vi "Action Update Ramp Rate-test-Caraya.vi"(8 "error in (no error)":errorcluster) -> (0 "error out":errorcluster)   [LabVIEW 2018]
doc: "The harness VI is executed for every test case. InstaCoverage passes the test case ID before the execution of the test case in the <b>test case ID</b> input and reads the <b>result</b> output after the execution. If the result is TRUE and no error happens during the execution, then the test case is evaluated as PASSED. If the result is false and no error happens during the execution, then the test case is evaluated as FAILED. Otherwise the test case is evaluated as ERROR.\n\nThe result of the test suite will be PASSED (FAILED) if all (at least one) test cases are PASSED (FAILED). If at least one test case in the test suite has the ERROR result, then the test suite will have ERROR result.\n\n<b>Note: </b>Don't change the connector pane of this VI.\n\nSee the Help Document for more information. (<b>Help</b> > <b>IncQuery Labs</b> > <b>InstaCoverage</b> > <b>InstaCoverage Help...</b>)"
uses:
  <vilib>/addons/_JKI Toolkits/Caraya/classes/Assert/Assert True.vi
  Libraries/Thermal Chamber Controller_DQMH/Thermal Chamber Controller_DQMH.lvlib
  <vilib>/addons/_JKI Toolkits/Caraya/classes/Test/Test.lvclass
  <vilib>/addons/_JKI Toolkits/Caraya/classes/Assert/Assert.lvclass
  Libraries/Thermal Chamber Response Simulator/Thermal Chamber Response Simulator.lvlib
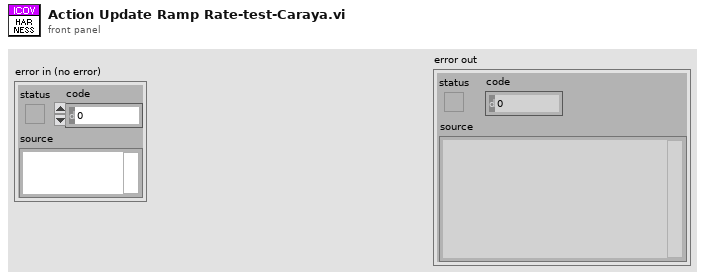
[diagram p1: front panel]
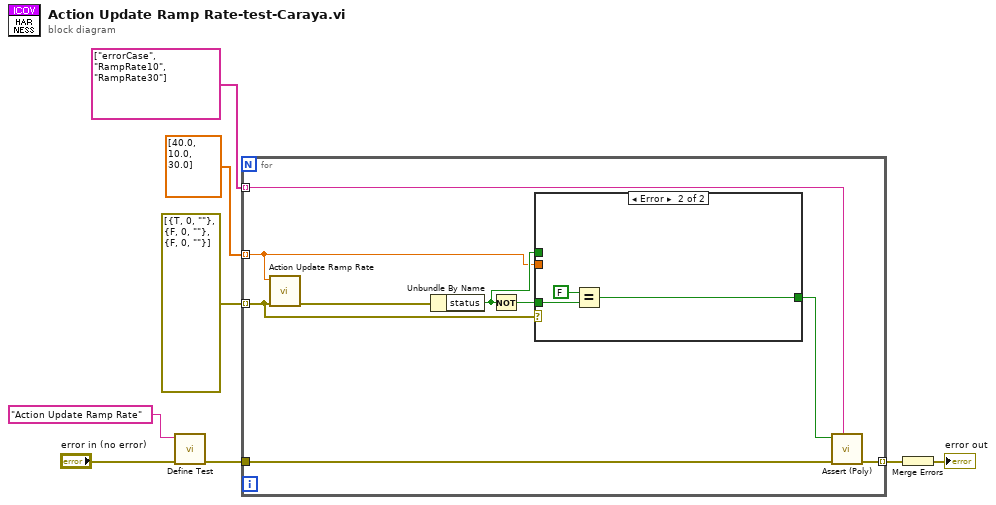
[diagram p0: block diagram]
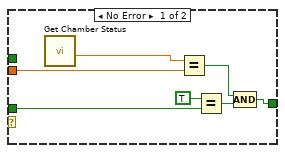
[diagram p2: hidden frame]
diagram:
  n1 = call <vilib>:"Define Test.vi"("error in (no error)"="error in (no error)", "Label (VI Title)"="Action Update Ramp Rate") -> ("error out"=w4:errorcluster)  [unwired: 9 in]
  n2 = for {
    tunnel: [w17] -> w6 mode=indexing
    tunnel: w4 -> [w16]
    tunnel: errorcluster[] [{"status"=TRUE, "code"=0, "source"=""}, {"status"=FALSE, "code"=0, "source"=""}, {"status"=FALSE, "code"=0, "source"=""}] -> [w15] mode=indexing
    tunnel: dbl[] [40.0, 10.0, 30.0] -> [w10] mode=indexing
    tunnel: string[] ["errorCase", "RampRate10", "RampRate30"] -> [w9] mode=indexing
    n3 = call "Action Update Ramp Rate.vi"("error in (no error)"=w15, "Temperature Ramp Rate"=w10) -> ("error out"=w14:errorcluster)  [unwired: 9 in]
    n4 = Unbundle By Name(w14) -> ("status"=w12:bool)
    n5 = Not(x=w12) -> (.not. x?=w11:bool)
    n6 = case shown="Error" w15 {
      tunnel: [w18 w26] -> w13
      tunnel: w12 -> [_ _]
      tunnel: w11 -> [w21 w25]
      tunnel: w10 -> [w19 _]
      frame No Error {
        n7 = call "Get Chamber Status.vi"() -> ("Ramp Rate (deg C / second)"=w20:dbl)  [unwired: 6 in, 5 out]
        n8 = Equal?(x=w20, y=w19) -> (x = y?=w23:bool)
        n9 = Equal?(x=TRUE, y=w21) -> (x = y?=w22:bool)
        n10 = Compound Arithmetic op=AND(w23, w22) -> (w18:bool)
      }
      frame Error {
        n11 = Equal?(x=FALSE, y=w25) -> (x = y?=w26:bool)
      }
    }
    n12 = call-poly <vilib>:"Assert (Poly).vi"("Label"=w9, "error in (no error)"=w16, "True?"=w13) -> ("error out"=w17:errorcluster)  [unwired: 8 in]
  }
  n13 = Merge Errors(w6) -> (→"error out":errorcluster)
